vi "TCP PC Engine.vi"() -> ()   [LabVIEW 2019]
uses:
  <userlib>/STM/Examples/Command Based Communication/subVIs/Stop FGV Commands.ctl
  <userlib>/STM/TCP/STM Get Connection Reference (TCP).vi
  <userlib>/STM/TCP/STM Read Message (TCP).vi
  <userlib>/STM/TCP/STM Write Message (TCP).vi
  <userlib>/STM/TCP/STM Read Meta Data (TCP Ref).vi
  Type Defs and Controls/Event Mode Control.ctl
  <userlib>/STM/_SubVIs/stm_MetaDataElement.ctl
panel:
  in  "Send Command":bool
  in  "Exit":bool
  in  "Target IP Address":string="192.168.1.200"
  out "Meta data":T1[](array[typedef])
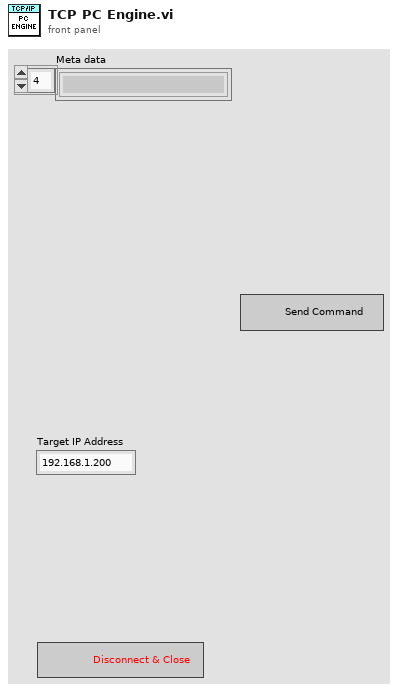
[diagram p1: front panel]
types:
  T1 = typedef "stm_MetaDataElement.ctl" = string
  T2 = typedef "Event Mode Control.ctl" = enum16{"Init", "Get", "Set", "Destroy"}
  T3 = typedef "Stop FGV Commands.ctl" = enum16{"Write", "Read", "Reset"}
  T4 = typedef "stm_TCP Connection Info.ctl" = cluster{"connection ID":refnum<k5>, "Meta data":T1[]}
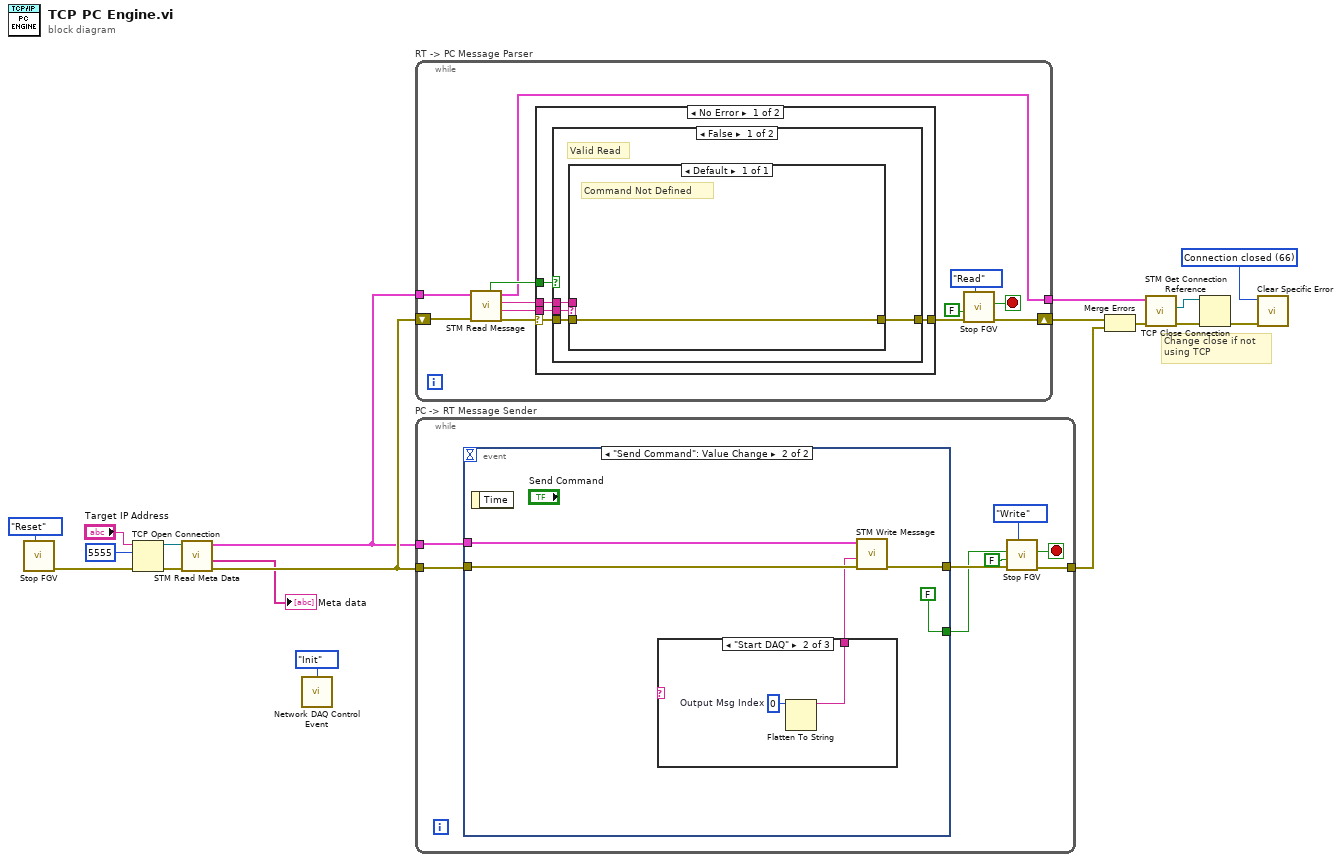
[diagram p0: block diagram]
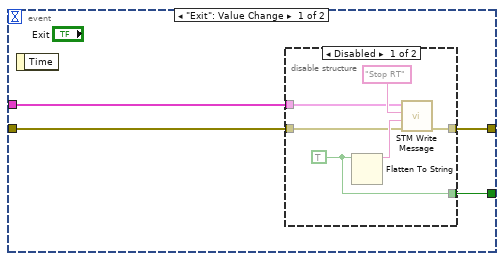
[diagram p2: hidden frame]
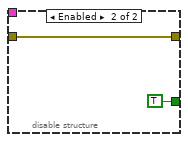
[diagram p3: hidden frame]
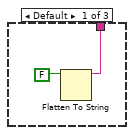
[diagram p4: hidden frame]
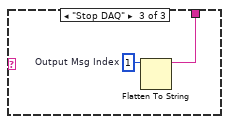
[diagram p5: hidden frame]
diagram:
  w15 = 66 items=["No Error", "Argument Error", "Memory Full", "Out of Zone", "End of File", "File Already Open", "Generic File IO Error", "File Not Found", "File Permission Error", "Disk Full", "Duplicate Path", "Too Many Files Open", "Not Enabled", "Resource File Not Found", "Cannot Add Resource", "Resource Not Found", "Image Not Found", "Image Memory Error", "Pen Does Not Exist", "Config Bad Type", "Config Token Not Found", "Config Parse Error", "Config Memory Error", "Bad External Code Format", "Bad External Code Offset", "External Code Not Present", "Null Window", "Destroy Window Mixup", "Null Menu", "Print Aborted", "Bad Print Record", "Print Driver Error", "Windows Error During Print", "Memory Error During Print", "Print Dialog Error", "Generic Print Error", "Invalid Device Refnum", "Device Not Found", "Device Parameter Error", "Device Unit Error", "Can't Open Device", "Device Call Aborted", "Generic Error", "Cancelled By User", "Object ID Too Low", "Object ID Too High", "Object Not In Heap", "Unknown Heap", "Bad DefProc ID", "DefProc Not In Table", "Message Out Of Range", "Null Method", "Unknown Message", "Manager Call Not Supported", "Bad address", "Connection In progress", "Connection timed out", "Connection is already in progress", "Network attribute not supported", "Network error", "Address in use", "System out of memory", "Connection aborted", "Connection refused", "Connection is not connected", "Connection is already connected", "Connection closed", "Initialize error (interapplication manager)", "Bad occurrence", "Wait on unbound occurrence handler", "Occurrence queue overflow", "Bad path", "Semaphore not signaled", "Unrecognized type (interapplication manager)"] ("1st Error to Convert")
  # "Change close if not using TCP"
  n1 = call <userlib>:"Stop FGV.vi"("Command"=Stop_FGV_Commands."Reset") -> ("error out"=w4:errorcluster)  [unwired: 3 in, 7 out]
  n2 = TCP Open Connection(address="Target IP Address", remote port or service name=u16 5555 ("remote port"), error in (no error)=w4) -> (connection ID=w5:refnum<k5>, error out=w6:errorcluster)  [unwired: 2 out]
  n3 = call-poly <userlib>:"STM Read Meta Data.vi"("error in"=w6, "connection ID"=w5) -> ("error out"=w17:errorcluster, "Meta data"=→"Meta data":T1[], "Connection Info Out"=w3:T4)  [unwired: 1 in, 6 out]
  n4 = call "Network DAQ Control Event.vi"("Mode (Set)"=Event_Mode_Control."Init") -> ()  [unwired: 13 in, 2 out]
  n5 = while "RT -> PC Message Parser" {
    tunnel: w3 -> [w30]
    shift-right: [w22] -> w9
    shift-left: w17 -> [w29]
    tunnel: [w20] -> w2
    stop <- w24 stop-if-true
    n6 = call-poly <userlib>:"STM Read Message.vi"("error in"=w29, "Connection Info"=w30) -> ("error out"=w25:errorcluster, "Name"=w28:T1, "data string"=w27:string, "Connection Info Out"=w20:T4, "Timed Out?"=w26:bool)  [unwired: 3 in, 2 out]
    n7 = case shown="No Error" w25 {
      selector: w25 -> [w32 w42]
      tunnel: w28 -> [w35 _]
      tunnel: w27 -> [w34 _]
      tunnel: w26 -> [w33 _]
      tunnel: [w31 w42] -> w23
      frame No Error {
        n8 = case shown="False" w33 {
          tunnel: w35 -> [w36 _]
          tunnel: w34 -> [w39 _]
          tunnel: w32 -> [w38 w41]
          tunnel: [w37 w41] -> w31
          frame False {
            # "Valid Read"
            n9 = case shown="Default" w36 {
              tunnel: w39 -> [_]
              tunnel: w38 -> [w40]
              tunnel: [w40] -> w37
              frame Default {
                # "Command Not Defined"
              }
            }
          }
          frame True {
            # "Valid Read, Timeout Present"
          }
        }
      }
      frame Error {
        # "TCP Error"
      }
    }
    n10 = call <userlib>:"Stop FGV.vi"("Command"=Stop_FGV_Commands."Read", "error in (no error)"=w23, "Stop on Error?"=FALSE) -> ("error out"=w22:errorcluster, "Latched Stop"=w24:bool)  [unwired: 1 in, 6 out]
  }
  n11 = while "PC -> RT Message Sender" {
    tunnel: w3 -> [w44]
    tunnel: w17 -> [w47]
    tunnel: [w49] -> w10
    stop <- w50 stop-if-true
    n12 = event shown="[1] \"Send Command\": Value Change" {
      selector: _ -> [_ _]
      dyn-events: _ -> [_ _]
      timeout: _ -> [_ _]
      tunnel: w44 -> [w51 w65]
      tunnel: w47 -> [w52 w66]
      tunnel: [w54 FALSE ("stop")] -> w45
      tunnel: [w53 w67] -> w46
      event "Exit": Value Change {
        n13 = event-data() -> ()  [unwired: 2 out]
        n14 = disable-structure shown="Disabled" {
          disable-tunnel: [w58 TRUE ("stop")] -> w54
          disable-tunnel: [w57 w62] -> w53
          disable-tunnel: w52 -> [w56 w62]
          disable-tunnel: w51 -> [w55 _]
          frame Disabled {
            w58 = TRUE ("stop")
            n15 = Flatten To String(anything=w58) -> (data string=w59:string)  [unwired: 2 in, 3 out]
            n16 = call-poly <userlib>:"STM Write Message.vi"("error in (no error)"=w56, "Data"=w59, "Name"="Stop RT", "Connection Info"=w55) -> ("error out"=w57:errorcluster)  [unwired: 1 in, 6 out]
          }
          frame Enabled {
          }
        }
      }
      event "Send Command": Value Change {
        n17 = event-data() -> ()  [unwired: 2 out]
        n18 = case shown="\"Start DAQ\"" {
          selector: _ -> [_ _ _]
          tunnel: [w68 w71 w72] -> w63
          frame Default {
            n19 = Flatten To String(anything=FALSE ("stop")) -> (data string=w68:string)  [unwired: 2 in, 3 out]
          }
          frame "Start DAQ" {
            w70 = u8 0  # Output Msg Index
            n20 = Flatten To String(anything=w70) -> (data string=w71:string)  [unwired: 2 in, 3 out]
          }
          frame "Stop DAQ" {
            w73 = u8 1  # Output Msg Index
            n21 = Flatten To String(anything=w73) -> (data string=w72:string)  [unwired: 2 in, 3 out]
          }
        }
        n22 = call-poly <userlib>:"STM Write Message.vi"("error in (no error)"=w66, "Data"=w63, "Connection Info"=w65) -> ("error out"=w67:errorcluster)  [unwired: 2 in, 6 out]
      }
    }
    n23 = call <userlib>:"Stop FGV.vi"("Command"=Stop_FGV_Commands."Write", "error in (no error)"=w46, "Stop on Error?"=FALSE, "Stop?"=w45) -> ("error out"=w49:errorcluster, "Latched Stop"=w50:bool)  [unwired: 6 out]
  }
  n24 = Merge Errors(w9, w10) -> (w8:errorcluster)
  n25 = call-poly <userlib>:"STM Get Connection Reference.vi"("error in"=w8, "Connection Info"=w2) -> ("error out"=w11:errorcluster, "connection ID out"=w12:refnum<k5>)  [unwired: 8 out]
  n26 = TCP Close Connection(connection ID=w12, error in (no error)=w11) -> (error out=w14:errorcluster)  [unwired: 2 out]
  n27 = call <userlib>:"Clear Specific Error.vi"("error in (no error)"=w14, "code"=w15) -> ()  [unwired: 10 out]
